vi "Launcher.vi"() -> ()   [LabVIEW 2009]
panel:
  in  "Control":string="Control\\Control.vi"
  in  "UI":string="UI\\Main_UI.vi"
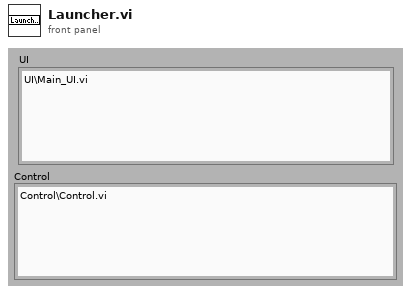
[diagram p1: front panel]
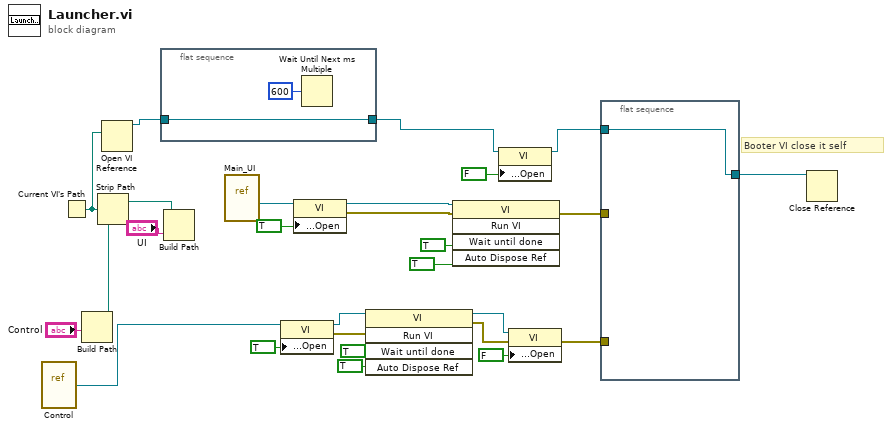
[diagram p0: block diagram]
diagram:
  # "Booter VI close it self"
  n1 = vi-ref "Control.vi"() -> (w10:refnum<vi>)
  n2 = Current VI's Path() -> (path=w26:path)
  n3 = Strip Path(path=w26) -> (stripped path=w19:path)  [unwired: 1 out]
  n4 = Build Path(base path=w19, name or relative path="Control") -> ()  [unwired: 1 out]
  n5 = Open VI Reference(vi path=w26) -> (vi reference=w4:refnum<vi>)  [unwired: 2 in, 4 out]
  n6 = flat-sequence {
    tunnel: w4 -> [w28]
    tunnel: [w28] -> w1
    frame #0 {
      n7 = Wait Until Next ms Multiple(millisecond multiple=u32 600) -> ()  [unwired: 1 out]
    }
  }
  n8 = Build Path(base path=w19, name or relative path="UI") -> ()  [unwired: 1 out]
  n9 = vi-ref "Main_UI.vi"() -> (w11:refnum<vi>)
  n10 = property class="VI"(reference=w10, "Front Panel.Open"=TRUE ("Front Panel Window:Open")) -> (reference out=w15:refnum<vi>, error out=w14:errorcluster)  [unwired: 1 in]
  n11 = property class="VI"(reference=w11, "Front Panel.Open"=TRUE ("Front Panel Window:Open")) -> (reference out=w21:refnum<vi>, error out=w22:errorcluster)  [unwired: 1 in]
  n12 = invoke class="VI" method="Run VI"(reference=w15, error in=w14, "Wait until done"=TRUE ("Wait Until Done"), "Auto Dispose Ref"=TRUE ("Auto Dispose Reference")) -> (reference out=w12:refnum<vi>, error out=w13:errorcluster)  [unwired: 1 in, 3 out]
  n13 = invoke class="VI" method="Run VI"(reference=w21, error in=w22, "Wait until done"=TRUE ("Wait Until Done"), "Auto Dispose Ref"=TRUE ("Auto Dispose Reference")) -> (error out=w6:errorcluster)  [unwired: 1 in, 4 out]
  n14 = property class="VI"(reference=w1, "Front Panel.Open"=FALSE ("Front Panel Window:Open")) -> (reference out=w2:refnum<vi>)  [unwired: 1 in, 1 out]
  n15 = property class="VI"(reference=w12, error in=w13, "Front Panel.Open"=FALSE ("Front Panel Window:Open")) -> (error out=w5:errorcluster)  [unwired: 1 out]
  n16 = flat-sequence {
    tunnel: w2 -> [w29]
    tunnel: [w29] -> w7
    tunnel: w6 -> [_]
    tunnel: w5 -> [_]
    frame #0 {
    }
  }
  n17 = Close Reference(reference=w7) -> ()  [unwired: 1 in, 1 out]
